vi "Destroy User Event - Stop.vi"(8 "error in":errorcluster, 11 "User Events":T1) -> (0 "error out":errorcluster)   [LabVIEW 2020, in "User Events.lvlib"]
doc: "Destroy the user event, even if there is an incoming error."
uses:
  User Events.lvlib
  User Events Refs--cluster.ctl
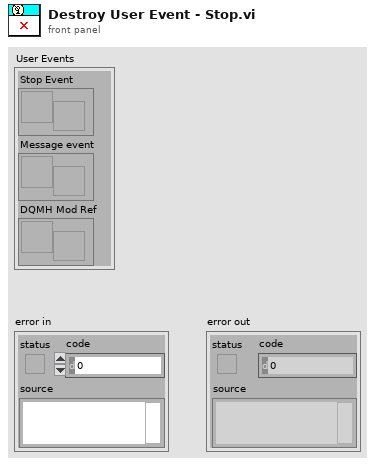
[diagram p1: front panel]
types:
  T1 = typedef "User Events.lvlib/User Events Refs--cluster.ctl" = cluster{"Stop Event":refnum<user-event>, "Message event ":refnum<user-event>, "DQMH Mod Ref":refnum<user-event>}
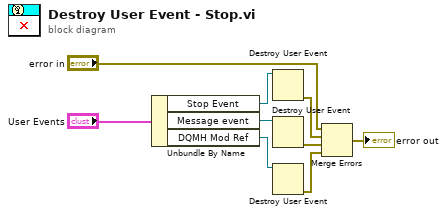
[diagram p0: block diagram]
diagram:
  n1 = Unbundle By Name("User Events") -> ("Stop Event"=w3:refnum<user-event>, "Message event"=w2:refnum<user-event>, "DQMH Mod Ref"=w1:refnum<user-event>)
  n2 = Destroy User Event(user event=w3) -> (error out=w7:errorcluster)  [unwired: 1 in]
  n3 = Destroy User Event(user event=w2) -> (error out=w6:errorcluster)  [unwired: 1 in]
  n4 = Destroy User Event(user event=w1) -> (error out=w5:errorcluster)  [unwired: 1 in]
  n5 = Merge Errors("error in", w7, w6, w5) -> (→"error out":errorcluster)
